vi "Set Output.vi"(6 "data":variant, 8 "error in (no error)":errorcluster, 9 "type":string, 10 "device":string, 11 "Device Manager in":refnum<class "Device Manager.lvclass">) -> (0 "error out":errorcluster, 2 "device not found?":bool, 3 "Device Manager out":refnum<class "Device Manager.lvclass">)   [LabVIEW 2023, in "Device Manager.lvclass"]
uses:
  Device Manager.lvclass
  Device Manager.lvclass/Device Manager.ctl
  Device/Device Messages/Output Action Msg/Output Action Msg.lvclass
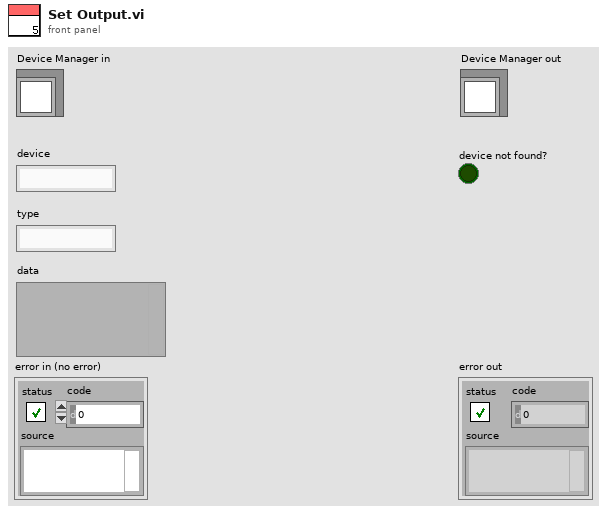
[diagram p1: front panel]
types:
  T1 = map{string, refnum<class "Message Enqueuer.lvclass">}
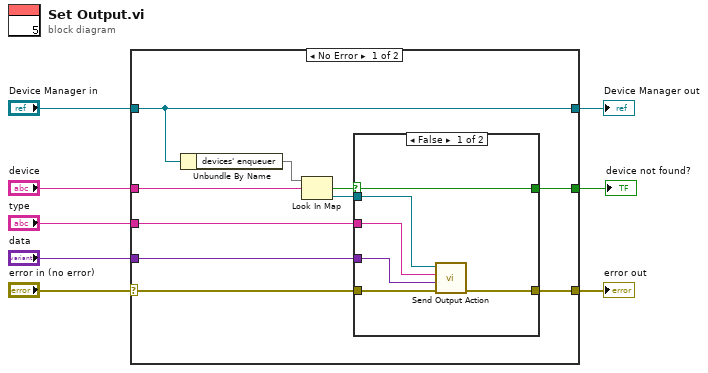
[diagram p0: block diagram]
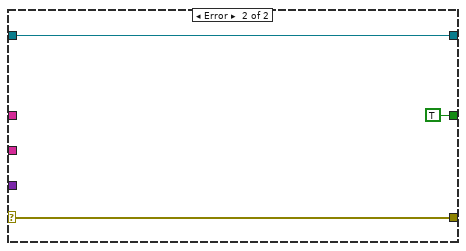
[diagram p3: hidden frame]
diagram:
  n1 = case shown="No Error" "error in (no error)" {
    selector: "error in (no error)" -> [w12 w29]
    tunnel: [w10 w29] -> w7
    tunnel: [w18 w28] -> w5
    tunnel: "Device Manager in" -> [w18 w28]
    tunnel: "device" -> [w16 _]
    tunnel: "type" -> [w14 _]
    tunnel: "data" -> [w13 _]
    tunnel: [w9 TRUE] -> w1
    frame No Error {
      n2 = Unbundle By Name(w18) -> ("devices' enqueuer"=w17:T1)
      n3 = Look In Map(map=w17, key=w16) -> (key not found?=w15:bool, value=w11:refnum<class "Message Enqueuer.lvclass">)  [unwired: 1 in]
      n4 = case shown="False" w15 {
        selector: w15 -> [w19 w25]
        tunnel: w14 -> [w22 _]
        tunnel: w13 -> [w23 _]
        tunnel: w12 -> [w24 w26]
        tunnel: w11 -> [w21 _]
        tunnel: [w20 w26] -> w10
        tunnel: [w19 w25] -> w9
        frame False {
          n5 = call "Send Output Action.vi"("error in (no error)"=w24, "data"=w23, "type"=w22, "Message Enqueuer"=w21) -> ("error out"=w20:errorcluster)  [unwired: 6 in, 1 out]
        }
        frame True {
        }
      }
    }
    frame Error {
    }
  }
  "error out" <- w7
  "Device Manager out" <- w5
  "device not found?" <- w1
